vi "ProcessName.vi"() -> (1 "process name":string)   [LabVIEW 2015, in "DeleteProcess.lvlib"]
uses:
  DeleteProcess.lvlib
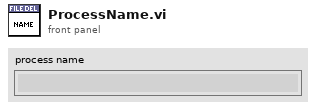
[diagram p1: front panel]
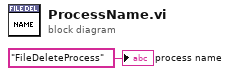
[diagram p0: block diagram]
diagram:
  "process name" <- "FileDeleteProcess" ("ProcessName")
